vi "Run Alicat Configuration.vi"(8 "error in (no error)":errorcluster, 11 "Alicat Device in":refnum<class "Alicat Device.lvclass">) -> (0 "error out":errorcluster, 1 "value":dbl, 2 "Accessors:controller_":bool, 3 "Alicat Device out":refnum<class "Alicat Device.lvclass">)   [LabVIEW 2015, in "Alicat Lib.lvlib" / "Alicat Device.lvclass"]
uses:
  Alicat Device.lvclass
  <vilib>/MSR Consulting, LLC/General Reuse/Session APIs/Serial/Serial Session.lvclass
  <vilib>/MSR Consulting, LLC/General Reuse/Session APIs/File Access/Config Data/Config Data.lvclass
  <vilib>/Utility/config.llb/NI_LVConfig.lvlib
  <vilib>/Utility/config.llb/Read Key (String).vi
  <vilib>/Utility/config.llb/Read Key (Double).vi
  <vilib>/MSR Consulting, LLC/General Reuse/Session APIs/_Session Fwk/Session - Root.lvclass
  <vilib>/ErrorRing/Error Ring.xnode
  <vilib>/MSR Consulting, LLC/General Reuse/Session APIs/Session Log/System Log.lvclass
  Data/Alicat Data.lvclass
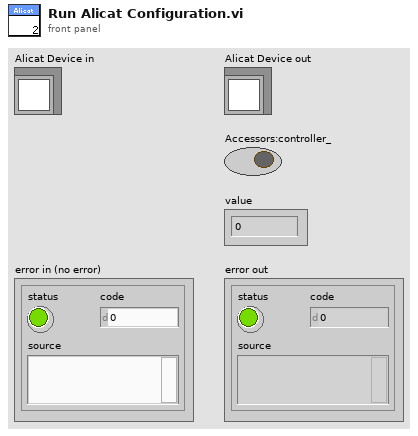
[diagram p1: front panel]
types:
  T1 = typedef "Serial Session.lvclass/Session Handle.ctl" = refnum<data-value>
  T2 = typedef "Config Data.lvclass/Config Session.ctl" = refnum<data-value>
  T3 = typedef "Session - Root.lvclass/Session Handle.ctl" = refnum<data-value>
  T4 = typedef "NI_LVConfig.lvlib/Config Data RefNum.ctl" = refnum<k1>
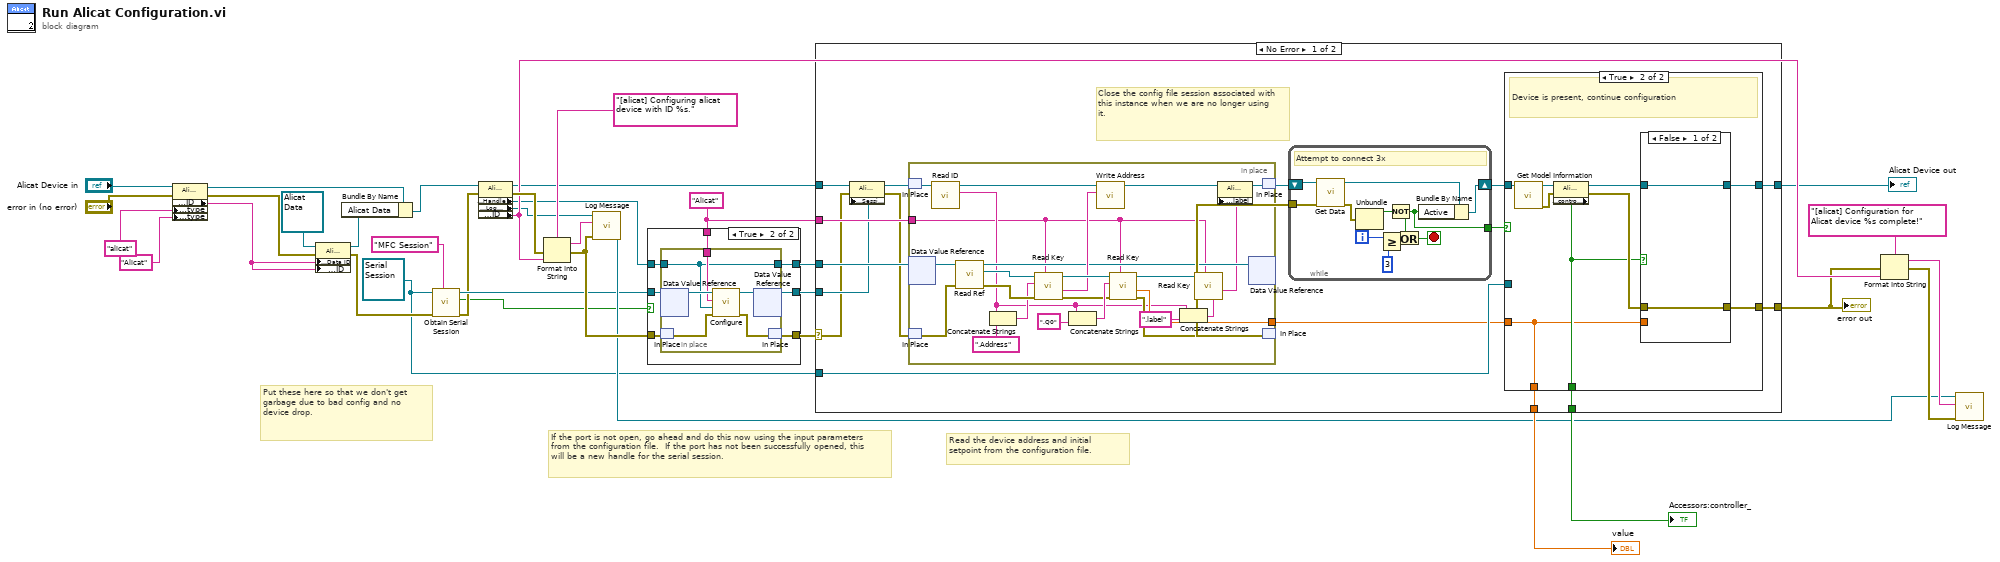
[diagram p0: block diagram]
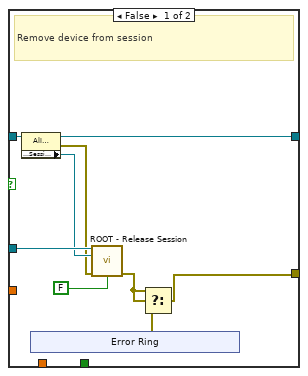
[diagram p2: hidden frame]
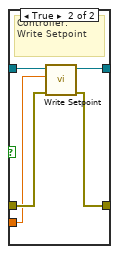
[diagram p3: hidden frame]
diagram:
  w9 = refnum<class "Serial Session.lvclass"> refnum ("Serial Session in")
  w7 = "Alicat" ("section")
  # "Put these here so that we don't get garbage due to bad config and no device drop."
  # "If the port is not open, go ahead and do this now using the input parameters from the configuration file.  If the port has not been successfully opened, this will be a new handle for the serial session."
  # "Read the device address and initial setpoint from the configuration file."
  n1 = property class="Alicat Device"(reference="Alicat Device in", error in="error in (no error)", "Accessors:type"="alicat" ("type"), "Accessors:type"="Alicat" ("section")) -> (reference out=w25:refnum<class "Alicat Device.lvclass">, error out=w28:errorcluster, "Accessors:ID"=w24:string)
  n2 = property class="Alicat Data"(reference=refnum<class "Alicat Data.lvclass"> refnum ("Alicat Lib.lvlib:Alicat Data"), error in=w28, "Accessors:Data ID"=w24, "Accessors:ID"=w24) -> (reference out=w27:refnum<class "Alicat Data.lvclass">, error out=w29:errorcluster)
  n3 = Bundle By Name(cluster=w25, "Alicat Data"=w27) -> (w26:refnum<class "Alicat Device.lvclass">)
  n4 = call <vilib>:"Obtain Serial Session.vi"("Session Name ()"="MFC Session", "error in"=w29, "Serial Session in"=w9) -> ("error out"=w5:errorcluster, "created new?"=w2:bool, "hSerial"=w8:T1)  [unwired: 6 in]
  n5 = property class="Alicat Device"(reference=w26, error in=w5) -> (reference out=w10:refnum<class "Alicat Device.lvclass">, error out=w30:errorcluster, "Accessors:Handle"=w4:T2, "Accessors:Log Session"=w14:T3, "Accessors:ID"=w22:string)
  n6 = Format Into String(format string="[alicat] Configuring alicat device with ID %s.", error in=w30, w22) -> (resulting string=w16:string, error out=w31:errorcluster)  [unwired: 1 in]
  n7 = call <vilib>:"Log Message.vi"("error in"=w31, "MSG In"=w16, "session in"=w14) -> ("session out"=w17:T3)  [unwired: 7 in, 1 out]
  n8 = case shown="True" w2 {
    tunnel: w8 -> [w39 w46]
    tunnel: w31 -> [w38 w42]
    tunnel: [w39 w45] -> w11
    tunnel: [w38 w44] -> w12
    tunnel: w4 -> [w37 w43]
    tunnel: [w37 w41] -> w6
    tunnel: w7 -> [_ w40]
    frame False {
    }
    frame True {
      n9 = in-place {
        in-place-border: w43 -> [w47]
        in-place-border: w40 -> [w48]
        in-place-border: [w47] -> w41
        n10 = in-place-dvr #1(w46) -> (w52:refnum<class "Serial Session.lvclass">)  [unwired: 1 out]
        n11 = in-place-match #2(w42) -> (w51:errorcluster)
        n12 = call <vilib>:"Configure.vi"("error in"=w51, "Config Handle"=w47, "section"=w48, "Serial Session in"=w52) -> ("error out"=w50:errorcluster, "Serial Session out"=w49:refnum<class "Serial Session.lvclass">)  [unwired: 6 in]
        n13 = in-place-dvr #1(w49) -> (w45:T1)  [unwired: 1 out]
        n14 = in-place-match #2(w50) -> (w44:errorcluster)
      }
    }
  }
  n15 = case shown="No Error" w12 {
    selector: w12 -> [w57 w131]
    tunnel: w6 -> [w69 _]
    tunnel: w7 -> [w68 _]
    tunnel: w9 -> [w67 _]
    tunnel: [w65 w131] -> w21
    tunnel: [w62 w132] -> w13
    tunnel: w10 -> [w61 w132]
    tunnel: w11 -> [w59 _]
    tunnel: [w54 _] -> w35
    tunnel: [w53 _] -> w36
    frame No Error {
      # "Close the config file session associated with this instance when we are no longer using it."
      n16 = property class="Alicat Device"(reference=w61, error in=w57, "Accessors:Session Handle"=w59) -> (reference out=w60:refnum<class "Alicat Device.lvclass">, error out=w58:errorcluster)
      n17 = in-place {
        in-place-border: w68 -> [w107]
        in-place-border: [w119] -> w63
        n18 = in-place-match #3(w60) -> (w117:refnum<class "Alicat Device.lvclass">)
        n19 = in-place-dvr #4(w69) -> (w130:refnum<class "Config Data.lvclass">)  [unwired: 1 out]
        n20 = in-place-match #5(w58) -> (w129:errorcluster)
        n21 = call "Read ID.vi"("Configurable Device in"=w117) -> ("ID"=w110:string, "Configurable Device out"=w116:refnum<class "Alicat Device.lvclass">)  [unwired: 8 in, 1 out]
        n22 = call <vilib>:"Read Ref.vi"("error in"=w129, "Config Data in"=w130) -> ("error out"=w127:errorcluster, "config data"=w128:T4, "Config Data out"=w118:refnum<class "Config Data.lvclass">)  [unwired: 7 in]
        n23 = Concatenate Strings(w110, ".Address" ("string")) -> (w125:string)
        n24 = call-poly <vilib>:"Read Key.vi"("section"=w107, "error in (no error)"=w127, "key"=w125, "refnum"=w128) -> ("error out"=w121:errorcluster, "value"=w120:string, "refnum out"=w124:T4)  [unwired: 4 in, 1 out]
        n25 = Concatenate Strings(w110, ".Q0" ("string")) -> (w122:string)
        n26 = call "Write Address.vi"("Address"=w120, "Alicat Device in"=w116) -> ("Alicat Device out"=w114:refnum<class "Alicat Device.lvclass">)  [unwired: 8 in, 1 out]
        n27 = call-poly <vilib>:"Read Key.vi"("section"=w107, "error in (no error)"=w121, "key"=w122, "refnum"=w124) -> ("error out"=w115:errorcluster, "value"=w119:dbl, "refnum out"=w109:T4)  [unwired: 4 in, 1 out]
        n28 = Concatenate Strings(w110, ".label" ("string")) -> (w111:string)
        n29 = call-poly <vilib>:"Read Key.vi"("section"=w107, "key"=w111, "refnum"=w109) -> ("value"=w108:string)  [unwired: 5 in, 3 out]
        n30 = property class="Alicat Device"(reference=w114, "Accessors:label"=w108) -> (reference out=w113:refnum<class "Alicat Device.lvclass">)  [unwired: 1 in, 1 out]
        n31 = in-place-dvr #4(w118) -> ()  [unwired: 2 out]
        n32 = in-place-match #3(w113) -> (w66:refnum<class "Alicat Device.lvclass">)
        n33 = in-place-match #5(w115) -> (w55:errorcluster)
      }
      n34 = while {
        tunnel: w55 -> [w101]
        shift-right: [w99] -> w64
        shift-left: w66 -> [w102]
        tunnel: [w98] -> w56
        i -> [w96]
        stop <- w103 stop-if-true
        # "Attempt to connect 3x"
        n35 = call-dynamic "Get Data.vi"("error in"=w101, "Alicat Device in"=w102) -> ("error out"=w97:errorcluster, "Alicat Device out"=w100:refnum<class "Alicat Device.lvclass">)  [unwired: 7 in, 1 out]
        n36 = Unbundle(w97) -> ("status"=w104:bool)  [unwired: 2 out]
        n37 = Greater Or Equal?(x=w96, y=3) -> (x >= y?=w105:bool)
        n38 = Not(x=w104) -> (.not. x?=w98:bool)
        n39 = Or(x=w98, y=w105) -> (x .or. y?=w103:bool)
        n40 = Bundle By Name(cluster=w100, "Active"=w98) -> (w99:refnum<class "Alicat Device.lvclass">)
      }
      n41 = case shown="True" w56 {
        tunnel: [w70 w87] -> w65
        tunnel: w67 -> [w78 _]
        tunnel: w64 -> [w76 w88]
        tunnel: w63 -> [_ w80]
        tunnel: [w75 w86] -> w62
        tunnel: [_ w81] -> w54
        tunnel: [_ w80] -> w53
        frame False {
          # "Remove device from session"
          n42 = property class="Alicat Device"(reference=w76) -> (reference out=w75:refnum<class "Alicat Device.lvclass">, error out=w73:errorcluster, "Accessors:Session Handle"=w74:T1)  [unwired: 1 in]
          n43 = xnode "Error Ring"() -> ("error out"=w71:errorcluster)
          n44 = call <vilib>:"ROOT - Release Session.vi"("OBJ - Session in"=w78, "Session Handle in"=w74, "error in (no error)"=w73, "force destroy? (F)"=FALSE) -> ("error out"=w72:errorcluster)  [unwired: 10 in, 1 out]
          n45 = Select(t=w72, s=w72, f=w71) -> (s? t:f=w70:errorcluster)
        }
        frame True {
          # "Device is present, continue configuration"
          n46 = call "Get Model Information.vi"("Alicat Device in"=w88) -> ("error out"=w82:errorcluster, "Alicat Device out"=w85:refnum<class "Alicat Device.lvclass">)  [unwired: 7 in, 2 out]
          n47 = property class="Alicat Device"(reference=w85, error in=w82) -> (reference out=w84:refnum<class "Alicat Device.lvclass">, error out=w83:errorcluster, "Accessors:controller_"=w81:bool)
          n48 = case shown="False" w81 {
            tunnel: w83 -> [w89 w94]
            tunnel: w84 -> [w90 w95]
            tunnel: w80 -> [_ w91]
            tunnel: [w89 w93] -> w87
            tunnel: [w90 w92] -> w86
            frame False {
            }
            frame True {
              # "Controller:\nWrite Setpoint"
              n49 = call "Write Setpoint.vi"("error in"=w94, "Setpoint"=w91, "Alicat Device in"=w95) -> ("error out"=w93:errorcluster, "Alicat Device out"=w92:refnum<class "Alicat Device.lvclass">)  [unwired: 6 in, 1 out]
            }
          }
        }
      }
    }
    frame Error {
    }
  }
  "value" <- w36
  "Accessors:controller_" <- w35
  "error out" <- w21
  "Alicat Device out" <- w13
  n50 = Format Into String(format string="[alicat] Configuration for Alicat device %s complete!", error in=w21, w22) -> (resulting string=w19:string, error out=w20:errorcluster)  [unwired: 1 in]
  n51 = call <vilib>:"Log Message.vi"("error in"=w20, "MSG In"=w19, "session in"=w17) -> ()  [unwired: 7 in, 2 out]
